vi "Control Panel.vi"() -> ()   [LabVIEW 2017]
uses:
  state-manager/State.ctl
  state-manager/Event.ctl
  <vilib>/Platform/TimedLoop/XDataNode/timing_clust.ctl
  <vilib>/Platform/TimedLoop/XDataNode/nitl_modes.ctl
  <vilib>/Platform/TimedLoop/XDataNode/wakeup.ctl
  <vilib>/myRIO/Instrument Drivers/Onboard IO/DIO/typedefs/DIO Reference.ctl
  <vilib>/myRIO/Common/Instrument Driver Framework/Utilities/typedefs/myRIO Generic Hardware Reference.ctl
  <vilib>/myRIO/Common/Instrument Driver Framework/Utilities/typedefs/Hardware Version Enum.ctl
  <vilib>/myRIO/Common/Instrument Driver Framework/Utilities/typedefs/myRIO v1.0 Reference.ctl
  <vilib>/myRIO/Common/Instrument Driver Framework/Utilities/typedefs/Generic FPGA Reference.ctl
  <vilib>/myRIO/Common/Instrument Driver Framework/myRIO v1.0/DIO/typedefs/DIO Channels List.ctl
  <vilib>/myRIO/Common/Instrument Driver Framework/myRIO v1.0/DIO/typedefs/DIO Channels Enum.ctl
  <vilib>/userdefined/High Color/nirio_resource_hc.ctl
  <vilib>/myRIO/Common/Instrument Driver Framework/Utilities/vis/Is FPGA Ref Available.vi
  <vilib>/myRIO/Common/Instrument Driver Framework/myRIO v1.0/DIO/vis/myRIO v1.1 Open DIO.vi
  <vilib>/myRIO/Instrument Drivers/Onboard IO/DIO/vis/Read.vi
  <vilib>/myRIO/Common/Instrument Driver Framework/Utilities/vis/Validate Channels.vi
  <vilib>/myRIO/Common/Instrument Driver Framework/myRIO v1.0/DIO/vis/myRIO v1.0 Reserve DIO.vi
  <vilib>/myRIO/Common/Instrument Driver Framework/myRIO v1.0/Resource Manager/vis/myRIO v1.0 Reserve Channel List.vi
  <vilib>/myRIO/Common/Instrument Driver Framework/myRIO v1.0/DIO/vis/myRIO v1.0 Build MUX Configuration DIO.vi
  <vilib>/myRIO/Common/Instrument Driver Framework/myRIO v1.0/Resource Manager/vis/myRIO v1.0 Reserve Channel.vi
  <vilib>/myRIO/Common/Instrument Driver Framework/myRIO v1.0/Resource Manager/vis/myRIO v1.0 Unreserve Channel.vi
  <vilib>/myRIO/Common/Instrument Driver Framework/myRIO v1.0/Resource Manager/vis/myRIO v1.0 Create Configuration List.vi
  <vilib>/myRIO/Common/Instrument Driver Framework/myRIO v1.0/Resource Manager/vis/myRIO v1.0 Build Mutex Name.vi
  Globals/Pose.vi
  Globals/Zig Zag Global.vi
  Globals/Gyro.vi
  <vilib>/Utility/VariantDataType/GetNumericInfo.vi
  <vilib>/Utility/error.llb/Error Cluster From Error Code.vi
  <vilib>/myRIO/Common/Instrument Driver Framework/myRIO v1.0/myRIO v1.1 Open.vi
  <vilib>/myRIO/Common/Instrument Driver Framework/Utilities/vis/IO Manager.vi
  <vilib>/myRIO/Common/Instrument Driver Framework/Utilities/vis/Configuration Manager.vi
  <vilib>/myRIO/Common/Instrument Driver Framework/myRIO v1.0/Resource Manager/vis/myRIO v1.0 Configure IO.vi
  <vilib>/myRIO/Common/Instrument Driver Framework/myRIO v1.0/myRIO v1.0 Close.vi
  <vilib>/myRIO/Common/Instrument Driver Framework/myRIO v1.0/DIO/vis/myRIO v1.0 Read DIO.vi
  Globals/Target Pose.vi
  Globals/Motor Speed Multiplier.vi
  <vilib>/Platform/TimedLoop/XDataNode/XDataNode.xnode
  <vilib>/myRIO/Express VI/Onboard IO/DI/DI Express VI.xnode
  <vilib>/myRIO/Instrument Drivers/Onboard IO/DIO/vis/myRIO DIO Open.xnode
  <vilib>/Platform/TimedLoop/XDataNode/XDNodeRunTimeDep.lvlib
  <vilib>/myRIO/Instrument Drivers/Onboard IO/DIO/DIO.lvlib
panel:
  out "Red Button Pressed":bool
  out "Nothing shat itself in test":bool
  out "Event list":T1[](array[typedef])=[enum."Black Tape Crossed", enum."Ramp Passed", enum."Black Tape Crossed"]
  out "State list":T2[](array[typedef])
  out "Event Queue":T1[](array[typedef])=[enum."Black Tape Crossed"]
  in  "Pass In Event":bool
  in  "Manual Pass In Event":T1=enum."Start Button Pressed"
  in  "Speed":T3={"\nMoving speed"=1.0296610169491527, "Turning speed limit"=1.0296610169491527} {"Turning speed limit" scale=0.0..4.5; "Moving speed" scale=0.0..4.5}
  out "Current State":T2
  in  "Target Wall Distance":dbl=250.0
  in  "Stop Motors":bool
  out "LIDAR Data":cluster{dbl[], dbl[]}(graph)
  in  "LIDAR display update period (ms)":i64=500
  out "Wall Left Indicator":bool=TRUE
  out "GYRO IS FUCKED":bool
  out "OH SHIT NO LIDAR DATA!!!":bool
  in  "OH SHIT, STOP":bool
  out "Gyro Bias":cluster{"X":dbl, "Y":dbl, "Z":dbl}={"X"=0.08609729920113632, "Y"=0.06396042865672143, "Z"=-0.2623400259994041}
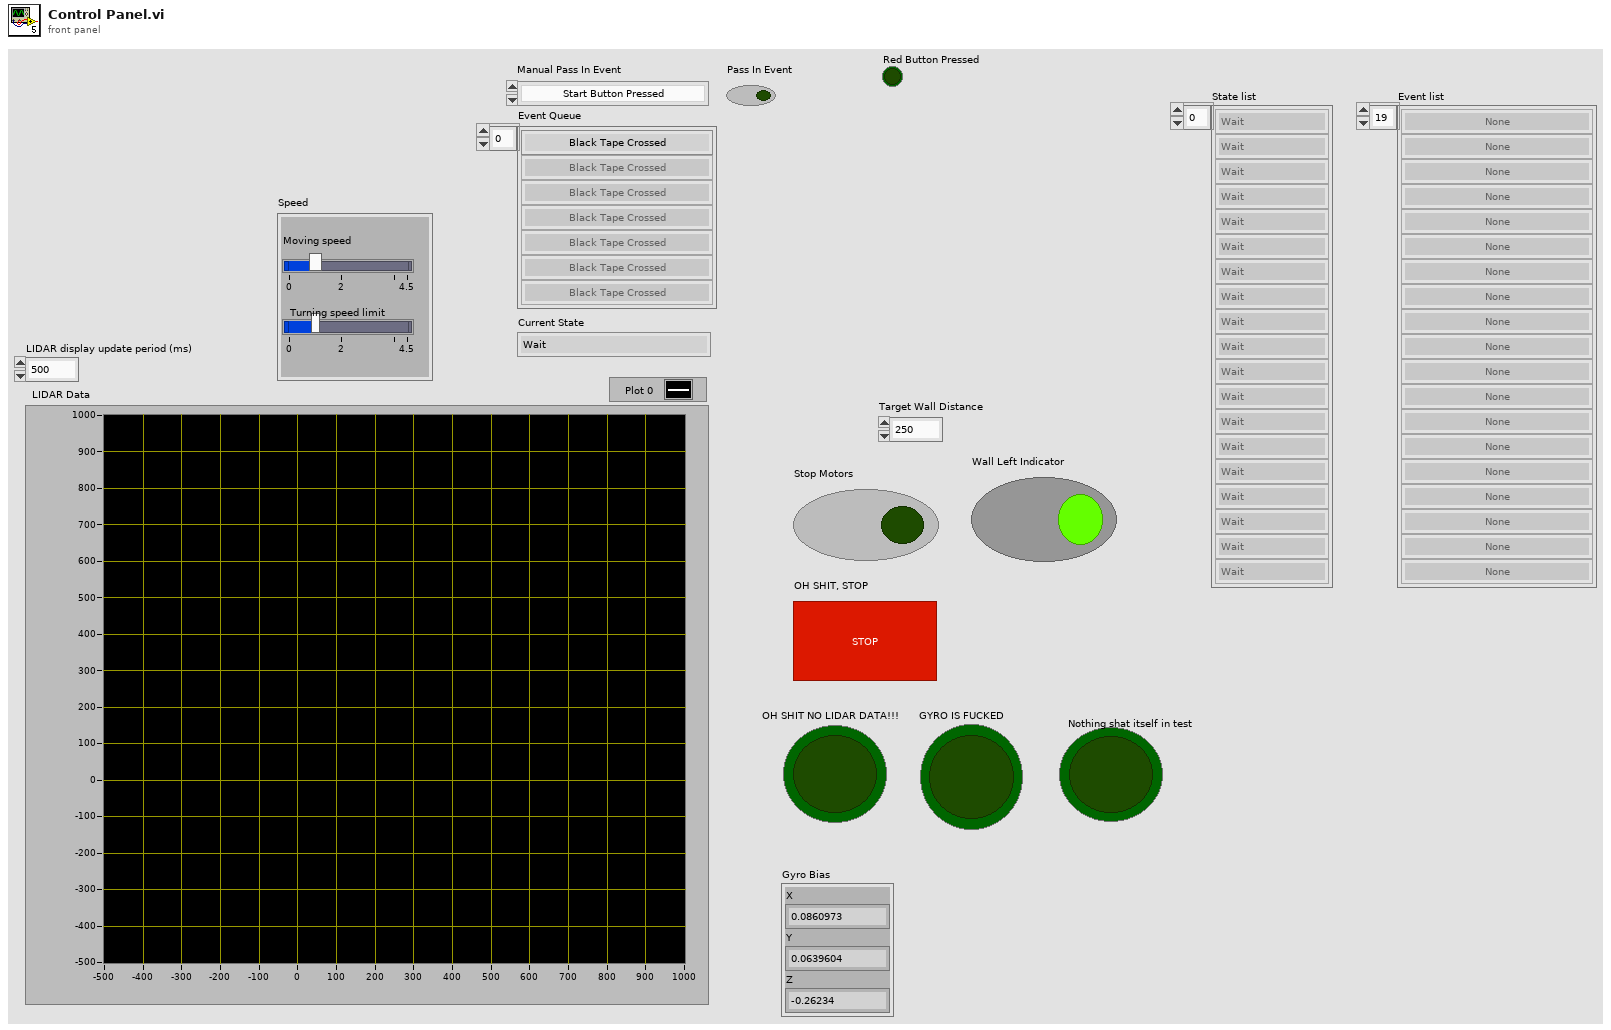
[diagram p1: front panel]
types:
  T1 = typedef "Event.ctl" = enum16{"None", "Zig Zag Finished", "Start Obstacle Avoidance", "Start Button Pressed", "Black & Yellow Tape Touched", "Black & Yellow Tape Passed", "Green Tape Crossed", "Red Tape Touched", "Rough Terrain Touched", "Black Tape Crossed", "Tape Edge Too Close", "Wall Too Close", "Rough Terrain Passed", "Ramp Passed", "Stop Button Pressed", "Recentered", "End Zone Wait Timed Out"}
  T2 = typedef "State.ctl" = enum16{"Wait", "Recenter", "Follow Wall", "Zig Zag", "Ramp", "Cross Rough Terrain", "Stagger Stop", "Obstacle Avoidance"}
  T3 = cluster{"\nMoving speed":dbl, "Turning speed limit":dbl}
  T4 = typedef "DIO.lvlib/DIO Reference.ctl" = cluster{"myRIO Reference":T5, "DIO Channels List":T9}
  T5 = typedef "myRIO Generic Hardware Reference.ctl" = cluster{"myRIO Model":T6, "myRIO Hardware Reference":T7}
  T6 = typedef "Hardware Version Enum.ctl" = enum16{"Unknown", "myRIO-1900", "myRIO-1950", "roboRIO", "NI ELVIS RIO CM"}
  T7 = typedef "myRIO v1.0 Reference.ctl" = cluster{"Generic FPGA Reference":T8, "Allow multiple opens":bool}
  T8 = typedef "Generic FPGA Reference.ctl" = refnum<k20>
  T9 = typedef "DIO Channels List.ctl" = T10[]
  T10 = typedef "DIO Channels Enum.ctl" = enum16{"Not Connected", "C/DIO0", "C/DIO1", "C/DIO2", "C/DIO3", "C/DIO4", "C/DIO5", "C/DIO6", "C/DIO7", "A/DIO0", "A/DIO1", "A/DIO2", "A/DIO3", "A/DIO4", "A/DIO5", "A/DIO6", "A/DIO7", "A/DIO8", "A/DIO9", "A/DIO10", "A/DIO11", "A/DIO12", "A/DIO13", "A/DIO14", "A/DIO15", "B/DIO0", "B/DIO1", "B/DIO2", "B/DIO3", "B/DIO4", "B/DIO5", "B/DIO6", "B/DIO7", "B/DIO8", "B/DIO9", "B/DIO10", "B/DIO11", "B/DIO12", "B/DIO13", "B/DIO14", "B/DIO15", "LED0", "LED1", "LED2", "LED3", "Button0", "DIO/DIO0", "DIO/DIO1", "DIO/DIO2", "DIO/DIO3", "DIO/DIO4", "DIO/DIO5", "DIO/DIO6", "DIO/DIO7", "DIO/DIO8", "DIO/DIO9", "SPI/CS0", "SPI/CS1", "SPI/CS2", "SPI/CS3", "LED RADIO (Green)", "LED RADIO (Red)", "LED COMM (Green)", "LED COMM (Red)", "LED MODE (Green)", "LED MODE (Red)"}
  T11 = typedef "nirio_resource_hc.ctl" = tag
  T12 = typedef "XDNodeRunTimeDep.lvlib/timing_clust.ctl" = cluster{"Expected End [f-1]":u64, "Actual End [f-1]":u64, "Finished Late? [f-1]":bool, "Expected End [i-1]":u64, "Actual End [i-1]":u64, "Finished Late? [i-1]":bool, "Expected Start [i]":u64, "Actual Start [i]":u64, "Expected Start [f]":u64, "Actual Start [f]":u64, "Source Name":string, "Structure Name":string, "Period":i64, "Deadline":i64, "Offset":i64, "Start":i64, "Priority":i32, "Timeout":i32, "Mode":T13, "Wakeup Reason":T14, "Error":errorcluster, "Source Type":string, "Secondary Source Type":string, "Global End Time":u64, "Global Start Time":u64, "Frame Duration":u64, "Iteration Duration":u64, "Assigned CPU":i32, "I/O Scan Engine Mode":u32}
  T13 = typedef "XDNodeRunTimeDep.lvlib/nitl_modes.ctl" = enum32{"No Change", "Process missed periods, maintain original phase", "Discard missed periods, maintain original phase", "Process missed periods, ignore original phase", "Discard missed periods, ignore original phase"}
  T14 = typedef "XDNodeRunTimeDep.lvlib/wakeup.ctl" = enum32{"Normal", "Aborted", "Asynchronous wakeup", "Timing source error", "Timed loop error", "Timeout"}
  T15 = typedef "IMAQdx.ctl" = refnum<k21>
  T16 = typedef "I2C.lvlib/I2C Reference.ctl" = cluster{"myRIO Reference":T5, "I2C Channels Enum":T17, "I2C Configuration":T18}
  T17 = typedef "I2C Channels Enum.ctl" = enum16{"Not Connected", "A/I2C", "B/I2C", "I2C/I2C"}
  T18 = typedef "I2C.lvlib/I2C Configuration.ctl" = cluster{"I2C Transfer Rate":T19}
  T19 = typedef "I2C.lvlib/I2C Transfer Rate.ctl" = enum16{"Standard mode (100 kbps)", "Fast mode (400 kbps)"}
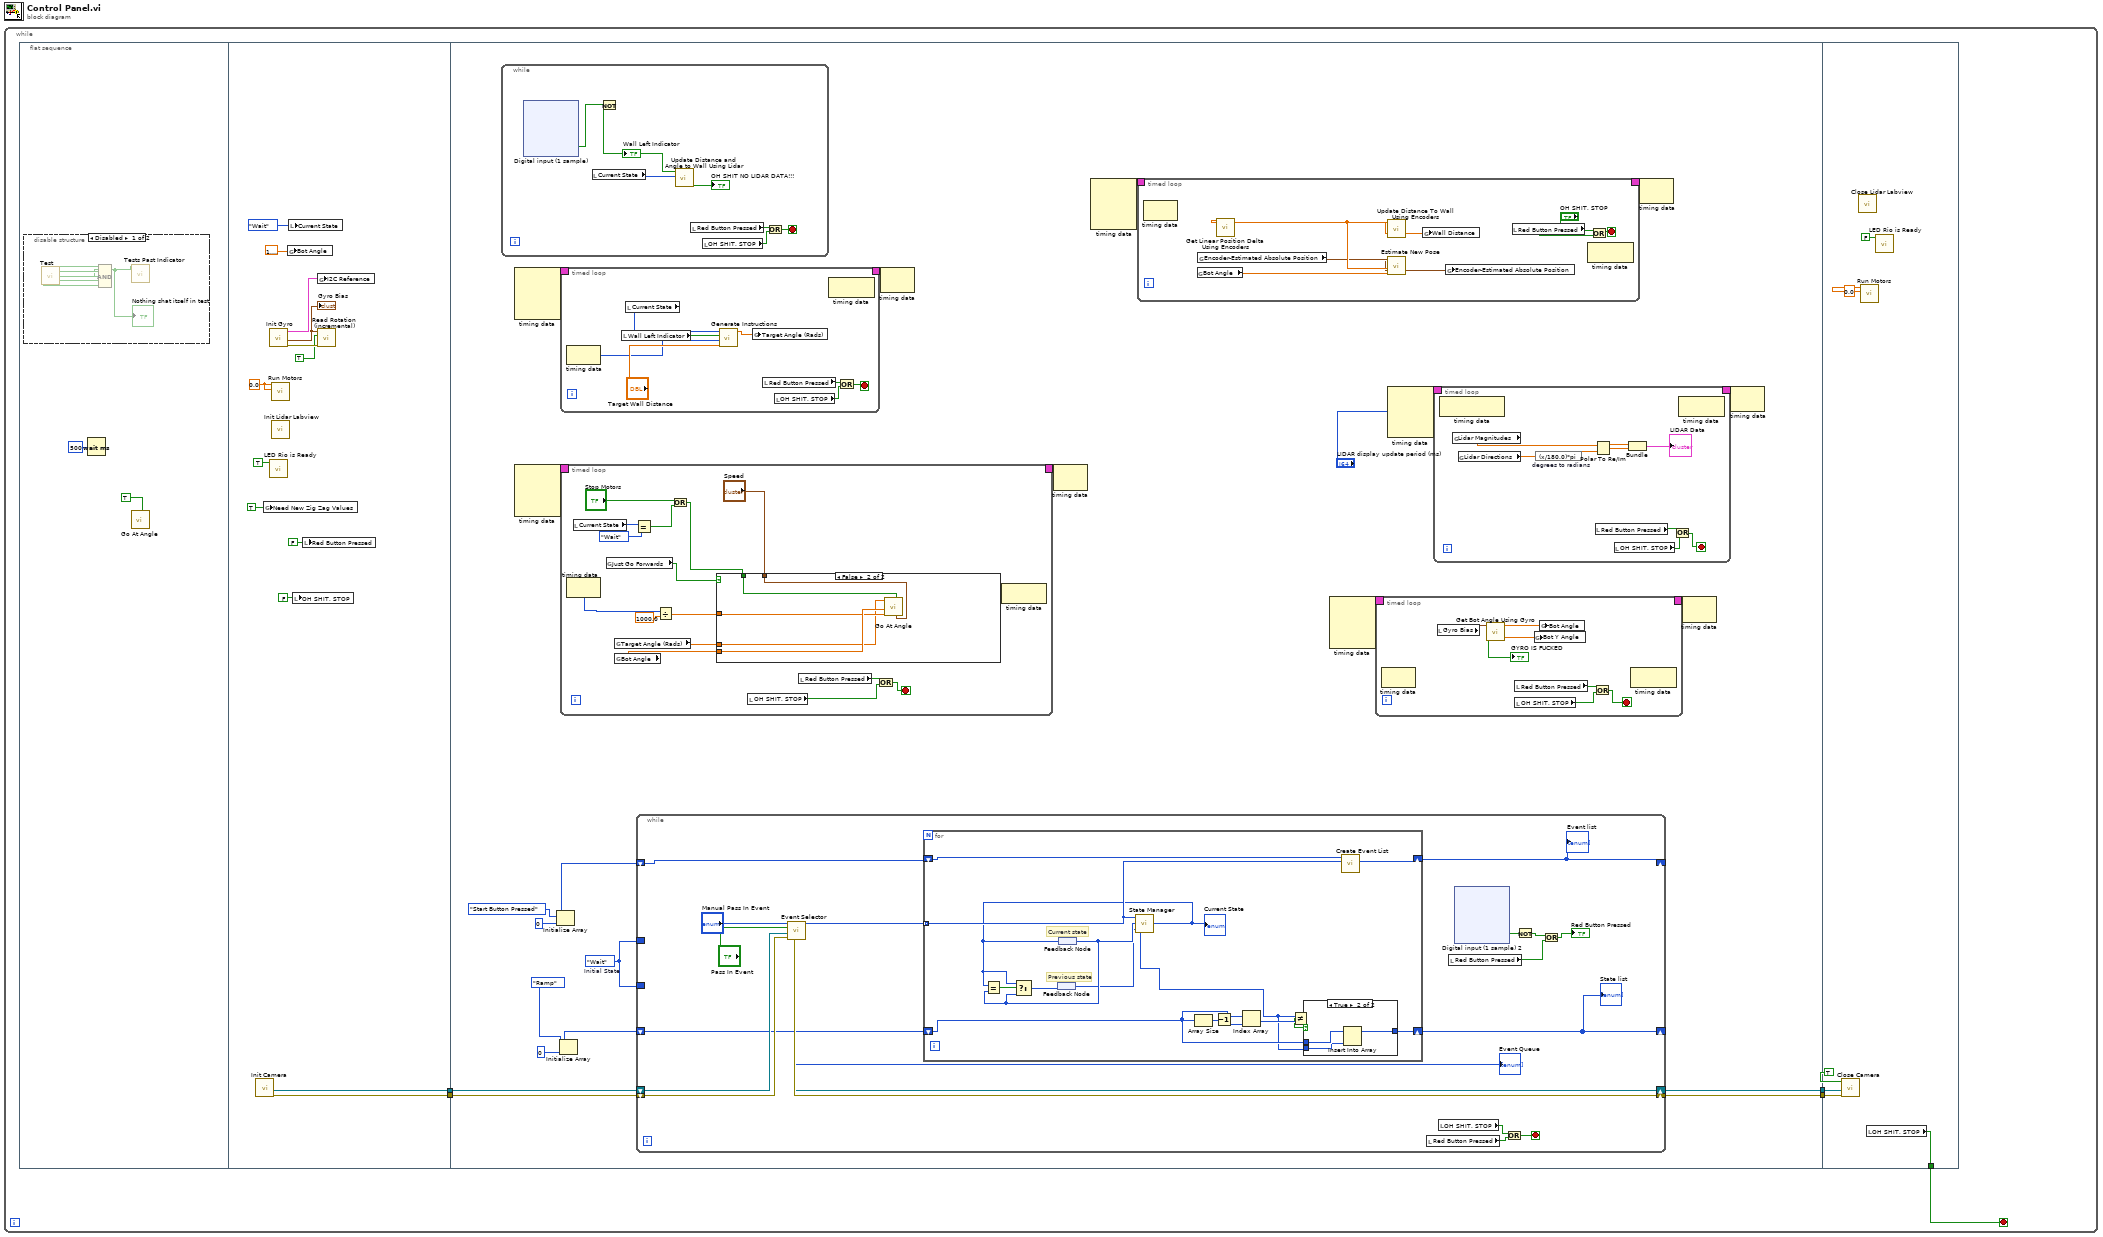
[diagram p0: block diagram]
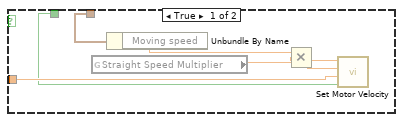
[diagram p4: hidden frame]
diagram:
  n1 = while {
    stop <- w1 stop-if-true
    n2 = flat-sequence {
      tunnel: [w21] -> w4
      tunnel: [w20] -> w5
      tunnel: w5 -> [w39]
      tunnel: [w38] -> w3
      tunnel: [w36] -> w2
      tunnel: w4 -> [w37]
      tunnel: w3 -> [w249]
      tunnel: w2 -> [w248]
      tunnel: [w244] -> w1
      frame #0 {
        n3 = disable-structure shown="Disabled" {
          frame Disabled {
            n4 = call "Test.vi"() -> ("Encoders Working\n(backwards)"=w13:bool, "Encoders Working\n(forwards)"=w12:bool, "Event Passed In Correctly"=w11:bool, "LIDAR Gets Data"=w10:bool, "Gyro Angle Correct 2"=w9:bool)  [unwired: 11 in]
            n5 = Compound Arithmetic op=AND(w13, w12, w11, w10, w9) -> (w8:bool)
            "Nothing shat itself in test" <- w8
            n6 = call "Tests Past Indicator.vi"("Test Past"=w8) -> ()  [unwired: 11 in]
          }
          frame Enabled {
          }
        }
        n7 = Wait (ms)(milliseconds to wait=u32 500) -> ()  [unwired: 1 out]
        n8 = call "Go At Angle.vi"("Stop motors"=TRUE) -> ()  [unwired: 10 in]
      }
      frame #1 {
        w26 = 0.0 ("Left motor speed (-1..1)")
        n9 = call "Init Camera.vi"() -> ("error out"=w21:errorcluster, "session out"=w20:T15)  [unwired: 9 in]
        n10 = global write "Zig Zag Global.vi" "Need New Zig Zag Values"(TRUE ("Zig Zag Finished")) -> ()
        n11 = call "Init Gyro.vi"() -> ("error out"=w16:errorcluster, "Gyro Bias"=w14:cluster{"X":dbl, "Y":dbl, "Z":dbl}, "I2C Ref Out"=w23:T16)  [unwired: 9 in]
        "Gyro Bias" <- w14
        n12 = call "LED Rio is Ready.vi"("Rio is ready"=TRUE) -> ()  [unwired: 11 in]
        n13 = call "Run Motors.vi"("Right motor side (-1..1)"=w26, "Left motor speed (-1..1)"=w26) -> ()  [unwired: 10 in]
        n14 = call "Init Lidar Labview.vi"() -> ()  [unwired: 11 in, 1 out]
        n15 = global write "Pose.vi" "Bot Angle"(1.5707963267948966) -> ()
        n16 = local write "Current State"(State."Wait" ("Current State")) -> ()
        n17 = local write "OH SHIT, STOP"(FALSE ("OH SHIT, STOP")) -> ()
        n18 = local write "Red Button Pressed"(FALSE ("Red Button Pressed")) -> ()
        n19 = global write "Gyro.vi" "I2C Reference"(w23) -> ()
        n20 = call "Read Rotation (incremental).vi"("error in (no error)"=w16, "reset"=TRUE, "Gyro bias"=w14) -> ()  [unwired: 7 in, 2 out]
      }
      frame #2 {
        w27 = State."Wait"  # Initial State
        n21 = while {
          stop <- w190 stop-if-true
          n22 = xnode "Digital input (1 sample)"() -> ("Switch for Left Right (A/DIO2 (Pin 15))"=w194:bool)  [unwired: 1 in, 1 out]
          n23 = local read "Current State"() -> (w195:T2)
          n24 = Not(x=w194) -> (.not. x?=w193:bool)
          "Wall Left Indicator" <- w193
          n25 = call "Update Distance and Angle to Wall Using Lidar.vi"("Current State"=w195, "Wall Left?"=w193) -> ("OH SHIT NO LIDAR DATA!!!"=→"OH SHIT NO LIDAR DATA!!!":bool)  [unwired: 9 in]
          n26 = local read "Red Button Pressed"() -> (w192:bool)
          n27 = local read "OH SHIT, STOP"() -> (w191:bool)
          n28 = Or(x=w192, y=w191) -> (x .or. y?=w190:bool)
        }
        n29 = node-c288() -> (w41:T12)  [unwired: 4 in]
        n30 = node-c288() -> (w35:T12)  [unwired: 4 in]
        n31 = Initialize Array(Event."Start Button Pressed" ("Event"), 0 ("dimension size")) -> (w28:T1[])
        n32 = Initialize Array(State."Ramp" ("y"), 0 ("dimension size")) -> (w31:T2[])
        n33 = timed-loop {
          timing: w41 -> [_]
          timing-out: [_] -> w40
          stop <- w152 stop-if-true
          n34 = node-c288() -> (w156:i64)  [unwired: 1 in]
          n35 = local read "Wall Left Indicator"() -> (w157:bool)
          n36 = local read "Current State"() -> (w155:T2)
          n37 = call "Generate Instructions.vi"("State"=w155, "Wall Left?"=w157, "dt"=w156, "Target Distance"="Target Wall Distance") -> ("Target Angle"=w154:dbl)  [unwired: 6 in]
          n38 = global write "Target Pose.vi" "Target Angle (Rads)"(w154) -> ()
          n39 = local read "Red Button Pressed"() -> (w153:bool)
          n40 = local read "OH SHIT, STOP"() -> (w151:bool)
          n41 = node-c288() -> ()  [unwired: 1 in, 1 out]
          n42 = Or(x=w153, y=w151) -> (x .or. y?=w152:bool)
        }
        n43 = timed-loop {
          timing: w35 -> [_]
          timing-out: [_] -> w34
          stop <- w125 stop-if-true
          n44 = node-c288() -> (w133:i64)  [unwired: 1 in]
          n45 = local read "Current State"() -> (w123:T2)
          n46 = global read "Pose.vi" "Just Go Forwards"() -> (w128:bool)
          n47 = global read "Target Pose.vi" "Target Angle (Rads)"() -> (w129:dbl)
          n48 = global read "Pose.vi" "Bot Angle"() -> (w132:dbl)
          n49 = Equal?(x=w123, y=State."Wait") -> (x = y?=w121:bool)
          n50 = Divide(x=w133, y=1000.0) -> (x/y=w131:dbl)
          n51 = Or(x="Stop Motors", y=w121) -> (x .or. y?=w120:bool)
          n52 = case shown="False" w128 {
            tunnel: w132 -> [_ w145]
            tunnel: w131 -> [w140 w144]
            tunnel: w120 -> [w139 w143]
            tunnel: "Speed" -> [w138 w142]
            tunnel: w129 -> [_ w141]
            frame True {
              n53 = global read "Motor Speed Multiplier.vi" "Straight Speed Multiplier"() -> (w135:dbl)
              n54 = Unbundle By Name(w138) -> ("Moving speed"=w137:dbl)
              n55 = Multiply(x=w137, y=w135) -> (x*y=w136:dbl)
              n56 = call "Set Motor Velocity.vi"("Disable motors"=w139, "dt"=w140, "Right motor speed rev/s"=w136, "Left motor speed rev/s"=w136) -> ()  [unwired: 8 in]
            }
            frame False {
              n57 = call "Go At Angle.vi"("Target Angle"=w141, "Bot Angle"=w145, "dt"=w144, "Stop motors"=w143, "Speed"=w142) -> ()  [unwired: 6 in]
            }
          }
          n58 = local read "OH SHIT, STOP"() -> (w126:bool)
          n59 = local read "Red Button Pressed"() -> (w127:bool)
          n60 = Or(x=w127, y=w126) -> (x .or. y?=w125:bool)
          n61 = node-c288() -> ()  [unwired: 1 in, 1 out]
        }
        n62 = while {
          shift-right: [w64] -> w36
          shift-left: w37 -> [w66]
          shift-right: [w63] -> w38
          shift-left: w39 -> [w65]
          shift-right: [w58] -> _
          shift-left: w31 -> [w59]
          shift-right: [w57] -> _
          shift-left: w28 -> [w56]
          border: w27 -> [_]
          border: w27 -> [_]
          stop <- w52 stop-if-true
          n63 = call "Event Selector.vi"("Error In"=w66, "Session In"=w65, "Pass In Event"="Pass In Event", "Manual Pass In Event"="Manual Pass In Event") -> ("Error Out"=w64:errorcluster, "Session Out"=w63:T15, "Event Queue"=w60:T1[])  [unwired: 5 in]
          "Event Queue" <- w60
          n64 = for {
            tunnel: w60 -> [w108] mode=indexing
            shift-right: [w110] -> w58
            shift-left: w59 -> [w111]
            shift-right: [w107] -> w57
            shift-left: w56 -> [w109]
            # "Previous state"
            # "Current state"
            n65 = feedback #1() -> (w103:T2)
            n66 = feedback #2() -> (w104:T2)
            n67 = call "State Manager.vi"("Previous State"=w103, "Current State"=w104, "Event"=w108) -> ("Next State"=w102:T2)
            "Current State" <- w102
            n68 = Equal?(x=w102, y=w104) -> (x = y?=w106:bool)
            n69 = Select(t=w102, s=w106, f=w104) -> (s? t:f=w105:T2)
            n70 = feedback-in #1(w105) -> ()
            n71 = feedback-in #2(w102) -> ()
            n72 = Array Size(array=w111) -> (size(s)=w115:i32)
            n73 = Decrement(x=w115) -> (x-1=w114:i32)
            n74 = Index Array(array=w111, index=w114) -> (element=w113:T2)
            n75 = Not Equal?(x=w102, y=w113) -> (x != y?=w112:bool)
            n76 = case shown="True" w112 {
              tunnel: w111 -> [w116 w119]
              tunnel: w102 -> [_ w118]
              tunnel: [w116 w117] -> w110
              frame False {
              }
              frame True {
                n77 = Insert Into Array(array=w119, new element=w118) -> (w117:T2[])  [unwired: 1 in]
              }
            }
            n78 = call "Create Event List.vi"("Event Outcome"=w108, "Array in"=w109) -> ("Array out"=w107:T1[])  [unwired: 9 in]
          }
          "State list" <- w58
          "Event list" <- w57
          n79 = local read "Red Button Pressed"() -> (w53:bool)
          n80 = local read "OH SHIT, STOP"() -> (w54:bool)
          n81 = local read "Red Button Pressed"() -> (w49:bool)
          n82 = xnode "Digital input (1 sample) 2"() -> ("A/DIO0 (Pin 11)"=w55:bool)  [unwired: 1 in, 1 out]
          n83 = Or(x=w54, y=w53) -> (x .or. y?=w52:bool)
          n84 = Not(x=w55) -> (.not. x?=w51:bool)
          n85 = Or(x=w51, y=w49) -> (x .or. y?=→"Red Button Pressed":bool)
        }
        n86 = node-c288(w40) -> ()  [unwired: 1 out]
        n87 = node-c288(w34) -> ()  [unwired: 1 out]
        n88 = node-c288() -> (w48:T12)  [unwired: 4 in]
        n89 = timed-loop {
          timing: w48 -> [_]
          timing-out: [_] -> w47
          stop <- w232 stop-if-true
          n90 = node-c288() -> ()  [unwired: 1 in, 1 out]
          n91 = global read "Pose.vi" "Bot Angle"() -> (w237:dbl)
          n92 = global read "Pose.vi" "Encoder-Estimated Absolute Position"() -> (w236:cluster{"X":dbl, "Y":dbl})
          n93 = call "Get Linear Position Delta Using Encoders.vi"() -> ("Change in Linear Position (mm)"=w238:dbl)  [unwired: 11 in]
          n94 = call "Update Distance To Wall Using Encoders.vi"("Linear Distance Travelled (mm)"=w238) -> ("Wall Distance"=w239:dbl)  [unwired: 10 in]
          n95 = call "Estimate New Pose.vi"("Bot Angle (rad)"=w237, "Linear Distance Travelled (mm)"=w238, "Current Absolute Position"=w236) -> ("Updated Absolute Position"=w235:cluster{"X":dbl, "Y":dbl})  [unwired: 8 in]
          n96 = global write "Pose.vi" "Wall Distance"(w239) -> ()
          n97 = global write "Pose.vi" "Encoder-Estimated Absolute Position"(w235) -> ()
          n98 = local read "Red Button Pressed"() -> (w233:bool)
          n99 = node-c288() -> ()  [unwired: 1 in, 1 out]
          n100 = Or(x="OH SHIT, STOP", y=w233) -> (x .or. y?=w232:bool)
        }
        n101 = node-c288() -> (w46:T12)  [unwired: 4 in]
        n102 = timed-loop {
          timing: w46 -> [_]
          timing-out: [_] -> w45
          stop <- w179 stop-if-true
          n103 = node-c288() -> ()  [unwired: 1 in, 1 out]
          n104 = local read "Gyro Bias"() -> (w183:cluster{"X":dbl, "Y":dbl, "Z":dbl})
          n105 = call "Get Bot Angle Using Gyro.vi"("Gyro bias"=w183) -> ("Y Rotation (rads)"=w182:dbl, "GYRO IS FUCKED"=→"GYRO IS FUCKED":bool, "Z Rotation (rads)"=w185:dbl)  [unwired: 7 in, 1 out]
          n106 = local read "Red Button Pressed"() -> (w181:bool)
          n107 = local read "OH SHIT, STOP"() -> (w180:bool)
          n108 = global write "Pose.vi" "Bot Y Angle"(w182) -> ()
          n109 = global write "Pose.vi" "Bot Angle"(w185) -> ()
          n110 = Or(x=w181, y=w180) -> (x .or. y?=w179:bool)
          n111 = node-c288() -> ()  [unwired: 1 in, 1 out]
        }
        n112 = node-c288("LIDAR display update period (ms)") -> (w44:T12)  [unwired: 3 in]
        n113 = timed-loop {
          timing: w44 -> [_]
          timing-out: [_] -> w43
          stop <- w164 stop-if-true
          n114 = node-c288() -> ()  [unwired: 1 in, 1 out]
          n115 = global read "Pose.vi" "Lidar Magnitudes"() -> (w172:dbl[])
          n116 = global read "Pose.vi" "Lidar Directions"() -> (w167:dbl[])
          n117 = expression code="(x/180.0)*pi" "degrees to radians"(w167) -> (w168:dbl[])
          n118 = Polar To Re/Im(2:w168, 3:w172) -> (0:w170:dbl[], 1:w171:dbl[])
          n119 = local read "Red Button Pressed"() -> (w166:bool)
          n120 = local read "OH SHIT, STOP"() -> (w165:bool)
          n121 = Bundle(w171, w170) -> (→"LIDAR Data":cluster{dbl[], dbl[]})  [unwired: 1 in]
          n122 = Or(x=w166, y=w165) -> (x .or. y?=w164:bool)
          n123 = node-c288() -> ()  [unwired: 1 in, 1 out]
        }
        n124 = node-c288(w47) -> ()  [unwired: 1 out]
        n125 = node-c288(w45) -> ()  [unwired: 1 out]
        n126 = node-c288(w43) -> ()  [unwired: 1 out]
      }
      frame #3 {
        w245 = 0.0
        n127 = call "Close Camera.vi"("error in"=w248, "Session In"=w249, "stop"=TRUE) -> ()  [unwired: 7 in, 2 out]
        n128 = call "Close Lidar Labview.vi"() -> ()  [unwired: 11 in, 1 out]
        n129 = call "Run Motors.vi"("Right motor side (-1..1)"=w245, "Left motor speed (-1..1)"=w245) -> ()  [unwired: 10 in]
        n130 = local read "OH SHIT, STOP"() -> (w244:bool)
        n131 = call "LED Rio is Ready.vi"("Rio is ready"=FALSE) -> ()  [unwired: 11 in]
      }
    }
  }
